vi "Modulation Table Load.vi"(8 "error in (no error)":errorcluster, 11 "VISA session in":refnum<visa-resource-name>) -> (0 "error out":errorcluster, 3 "VISA session out":refnum<visa-resource-name>)   [LabVIEW 2011, in "Magna PSU.lvlib"]
uses:
  Magna PSU.lvlib
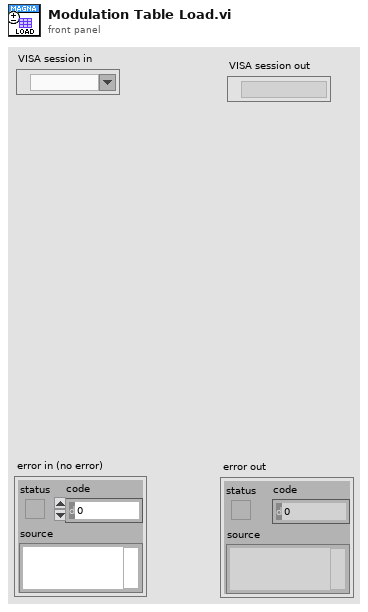
[diagram p1: front panel]
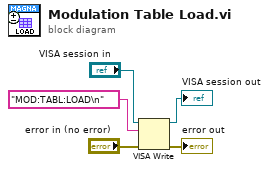
[diagram p0: block diagram]
diagram:
  n1 = VISA Write(VISA resource name="VISA session in", write buffer="MOD:TABL:LOAD\n", error in (no error)="error in (no error)") -> (VISA resource name out=→"VISA session out":refnum<visa-resource-name>, error out=→"error out":errorcluster)  [unwired: 1 out]
